vi "writeU64FIFO.vi"(8 "error in (no error)":errorcluster, 9 "Timeout":i32, 10 "Data":u64[](array[numeric]), 11 "MyHealthAndStatusWriteFIFO in":refnum<class "MyHealthAndStatusWriteFIFO.lvclass">) -> (0 "error out":errorcluster, 2 "ElementsRemaining":u32, 3 "MyHealthAndStatusWriteFIFO out":refnum<class "MyHealthAndStatusWriteFIFO.lvclass">)   [LabVIEW 2016, in "MyHealthAndStatusWriteFIFO.lvclass"]
uses:
  MyHealthAndStatusWriteFIFO.lvclass
  MyHealthAndStatusWriteFIFO.lvclass/MyHealthAndStatusWriteFIFO.ctl
  <vilib>/Utility/error.llb/Error Cluster From Error Code.vi
  <vilib>/rvi/errors/niLvFpgaAdjustHostInterfaceError.vi
  <vilib>/rvi/interface/nirviMethod/nirviMethod.xnode
  <vilib>/FPGAPlugInAG/Dynamic/niLvFpga_WriteFifo_Dynamic.vi
  <vilib>/rvi/errors/niLvFpgaMergeErrorWithErrorCode.vi
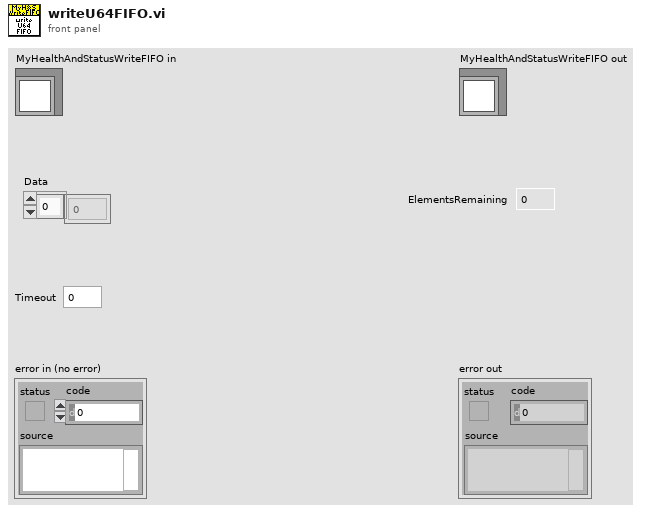
[diagram p1: front panel]
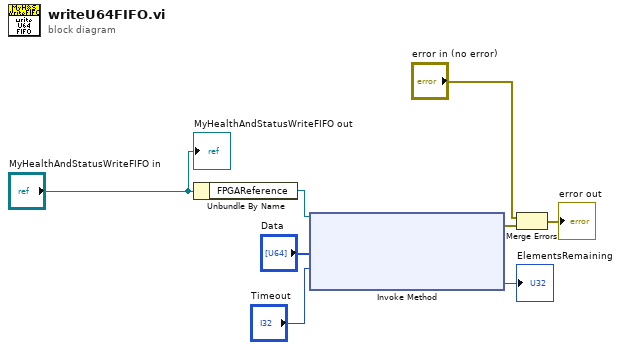
[diagram p0: block diagram]
diagram:
  n1 = Unbundle By Name("MyHealthAndStatusWriteFIFO in") -> ("FPGAReference"=w8:refnum<k20>)
  n2 = xnode "Invoke Method"("FPGA VI Reference In"=w8, "Data"="Data", "Timeout (ms)"="Timeout") -> ("error out"=w4:errorcluster, "Empty Elements Remaining"=→"ElementsRemaining":u32)  [unwired: 1 in, 1 out]
  n3 = Merge Errors("error in (no error)", w4) -> (→"error out":errorcluster)
  "MyHealthAndStatusWriteFIFO out" <- "MyHealthAndStatusWriteFIFO in"
